vi "一体站流程平行样自动启动.vi"(9 "参数":T1={"是否启用仪器"=FALSE, "CODMn"={"启动测量模式"={"测量模式"=enum."水样测量"}, "确定按钮"=TRUE}, "启动模块"={"氨氮1"=FALSE, "总磷1"=FALSE, " COD1"=FALSE}, "常规启动"=FALSE, "直接启动"=FALSE}) -> ()   [LabVIEW 2016, in "质控单元.lvlib"]
uses:
  PLC/PLC.lvlib
panel:
  out "COD平行样测完标志":bool
  out "氨氮总磷平行样测完标志":bool
  out "枚举 2":enum16{"初始化", "采配水启动", "等待", "配水", "排水", "结束"}(ring)
  out "枚举":enum16{"初始化", "采配水启动", "等待", "配水", "排水", "结束"}(ring)
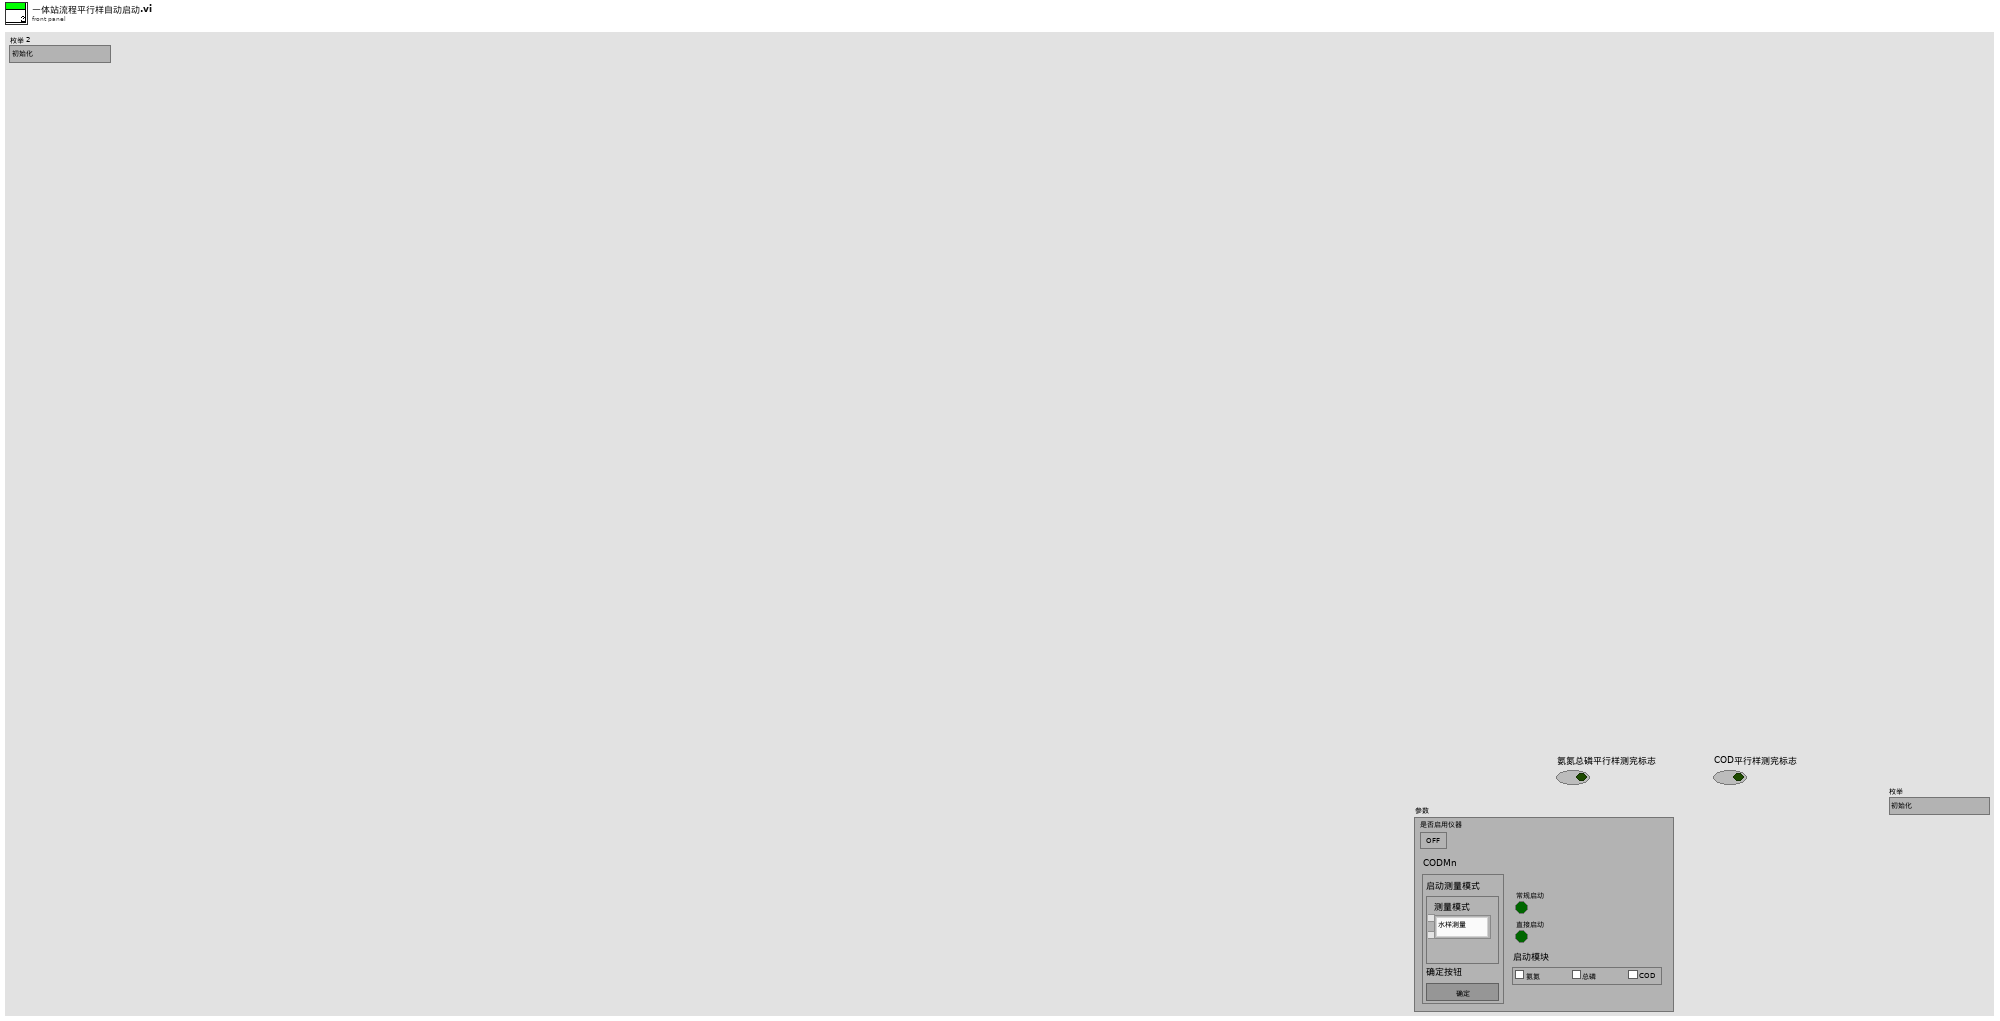
[diagram p1: front panel]
types:
  T1 = cluster{"是否启用仪器":bool, "CODMn":cluster{"启动测量模式":cluster{"测量模式":enum16{"水样测量", "标样核查", "加标回收", "平行样", "校零", "校标"}}, "确定按钮":bool}, "启动模块":cluster{"氨氮1":bool, "总磷1":bool, " COD1":bool}, "常规启动":bool, "直接启动":bool}
  T2 = cluster{"命令":string, cluster{"starting address":u16, "holding register value":u16}}
  T3 = cluster{"R0":i16, "R1":i16, "R2":i16, "R3":i16, "R4":i16, "R5":i16, "R6":i16, "R7":i16, "R8":i16, "R9":i16, "R10":i16, "R11":i16, "R12":i16, "R13":i16, "R14":i16, "R15":i16, "R16":i16, "R17":i16, "R18":i16, "R19":i16, "R20":i16, "R21":i16, "R22":i16, "R23":i16, "R24":i16, "R25":i16, "R26":i16, "R27":i16, "R28":i16, "R29":i16, "R30":i16, "R31":i16, "R32":i16, "R33":i16, "R34":i16}
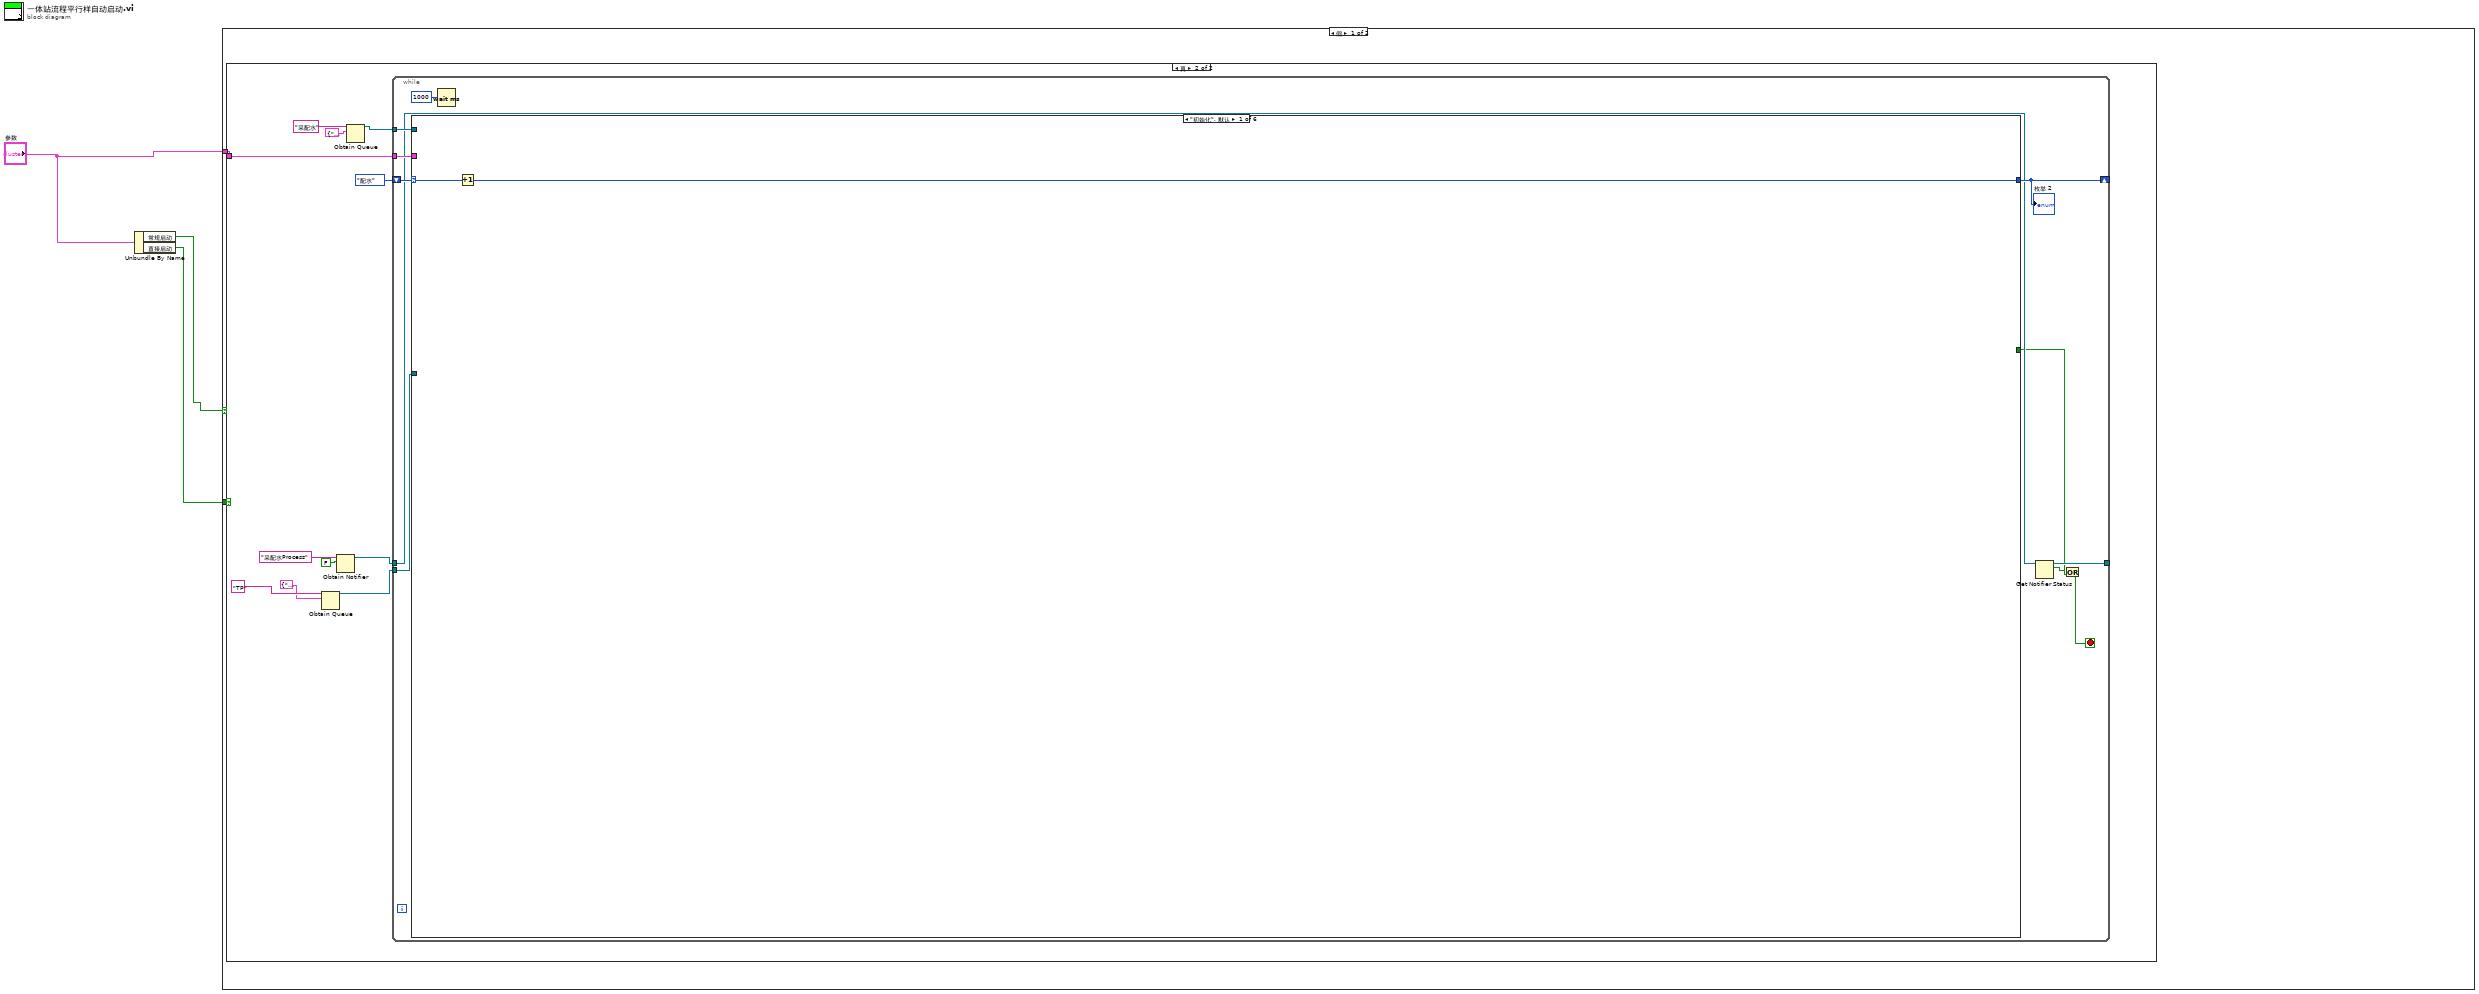
[diagram p0: block diagram]
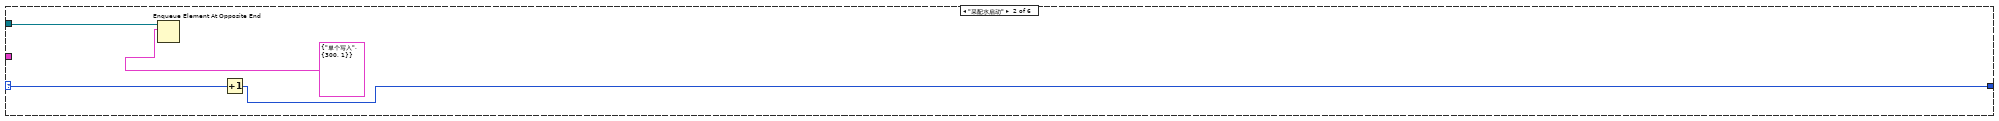
[diagram p3: hidden frame]
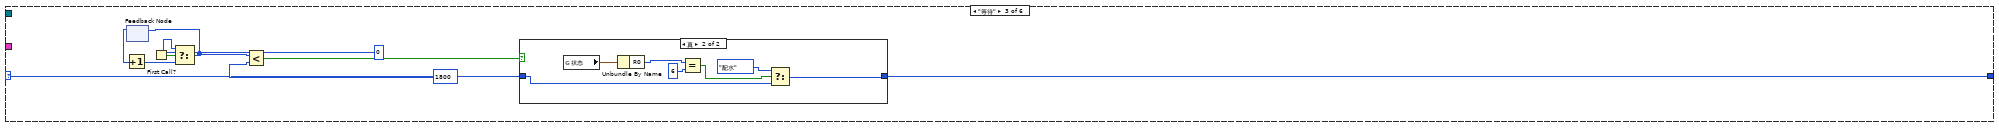
[diagram p4: hidden frame]
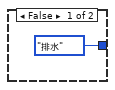
[diagram p5: hidden frame]
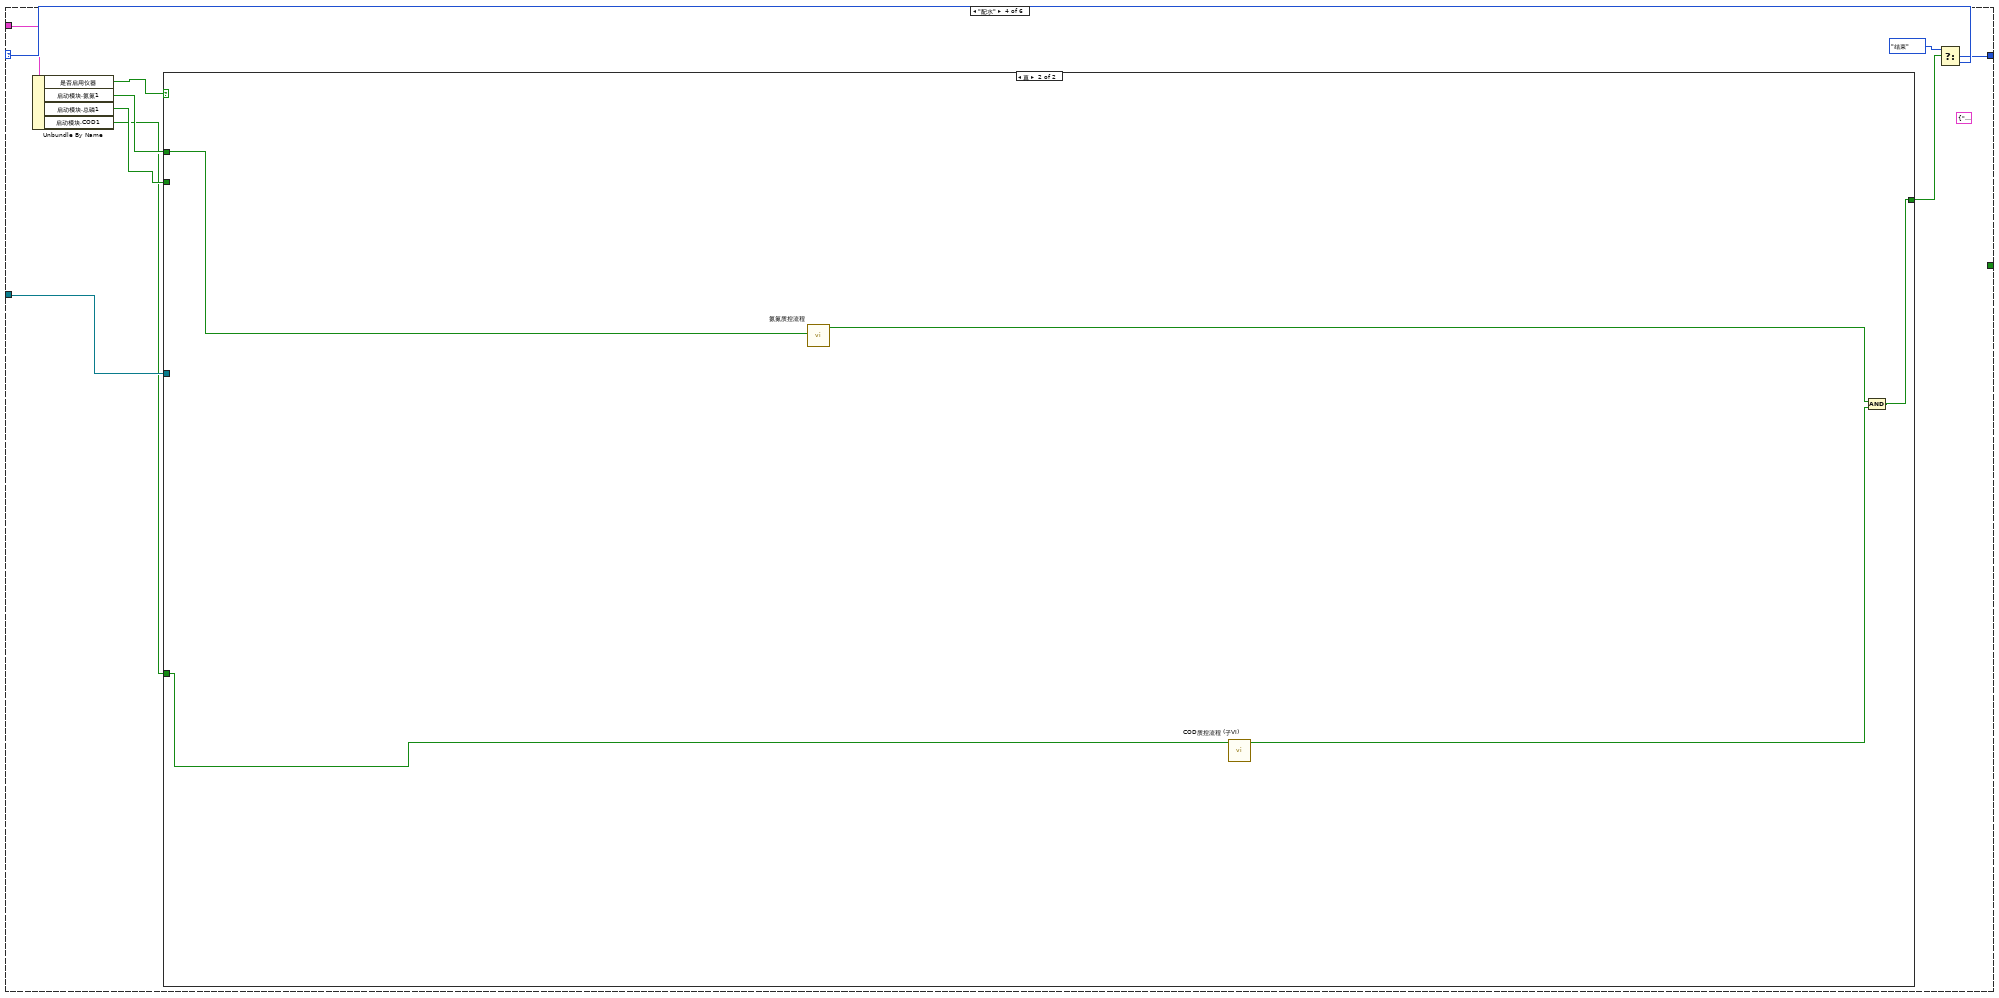
[diagram p6: hidden frame]
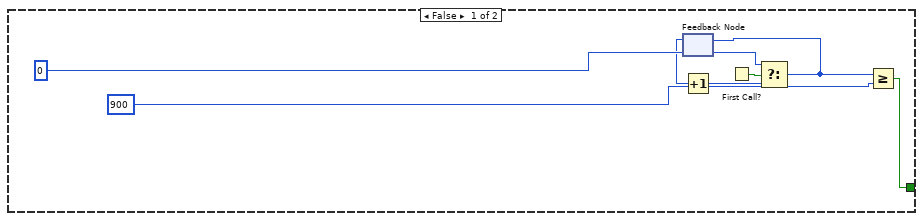
[diagram p7: hidden frame]
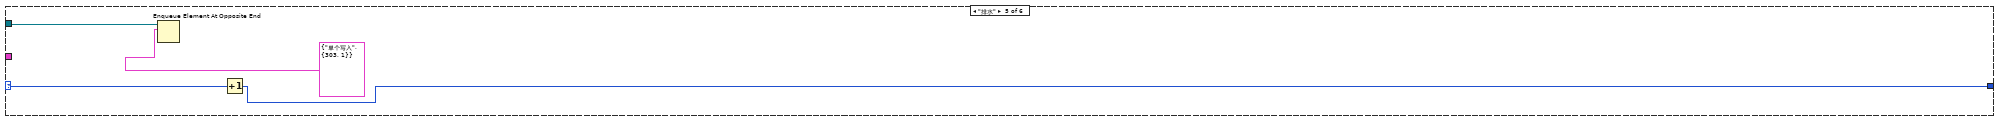
[diagram p8: hidden frame]
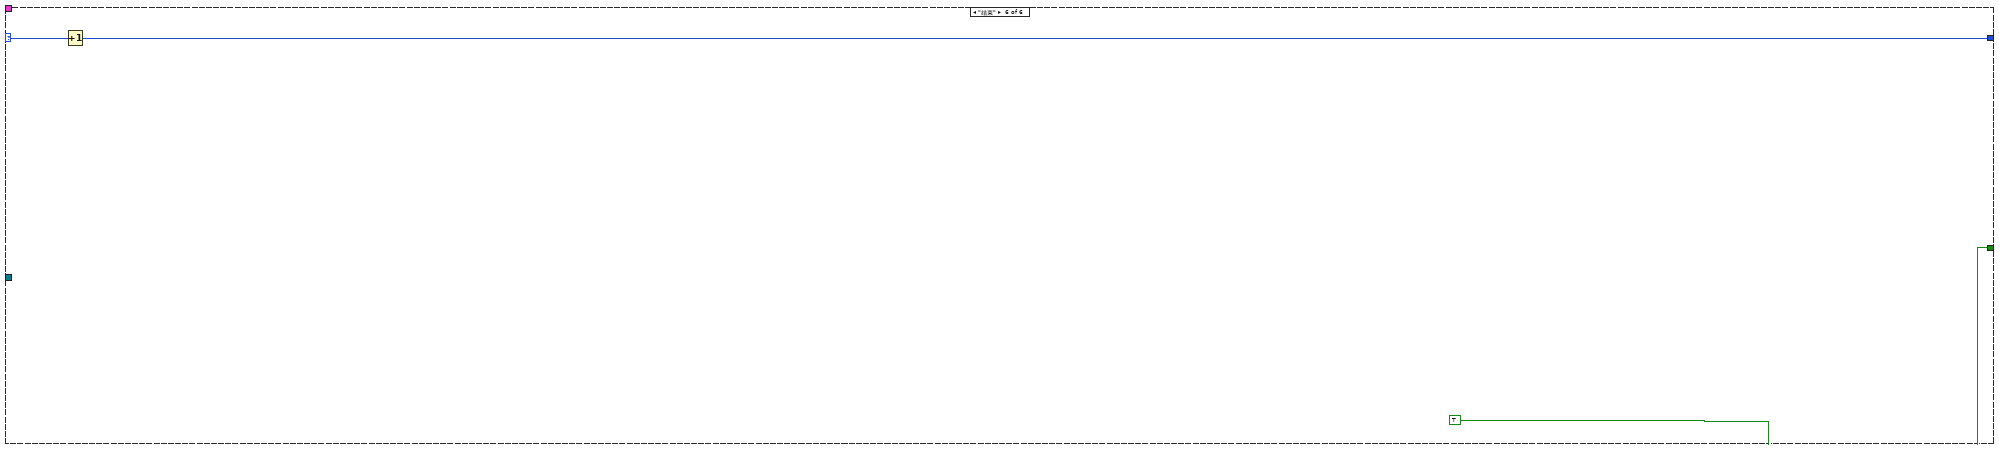
[diagram p9: hidden frame]
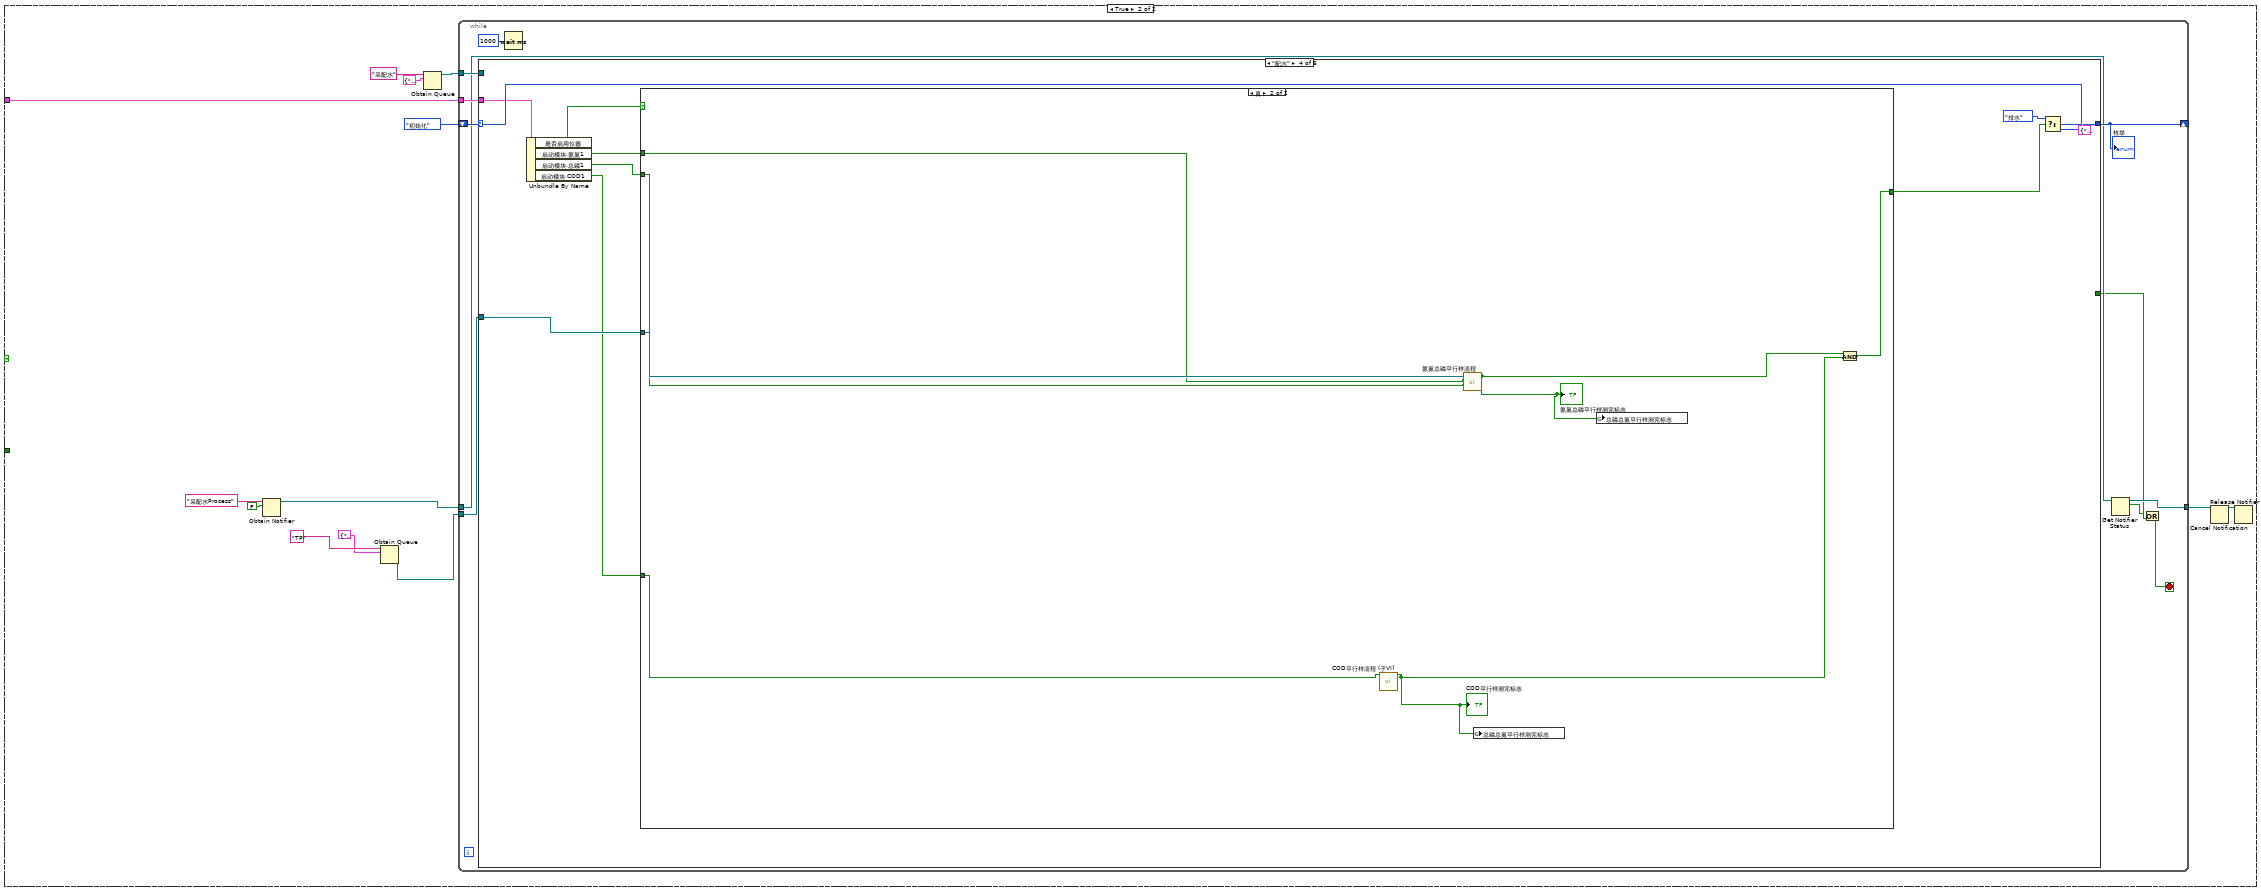
[diagram p10: hidden frame]
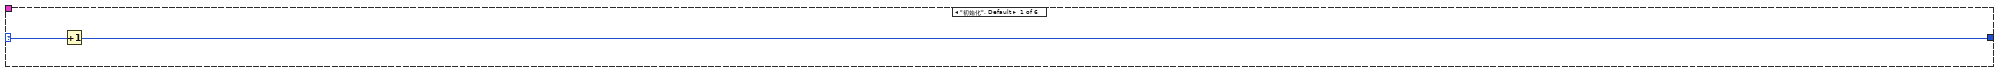
[diagram p11: hidden frame]
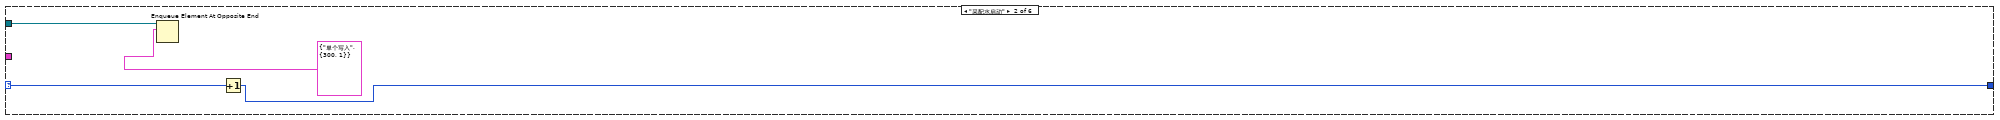
[diagram p12: hidden frame]
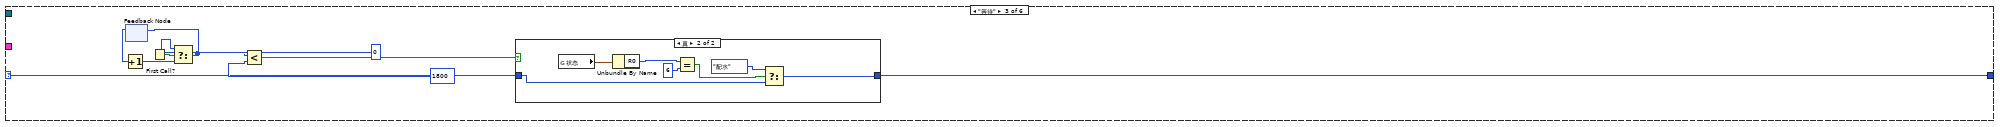
[diagram p13: hidden frame]
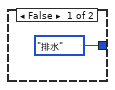
[diagram p14: hidden frame]
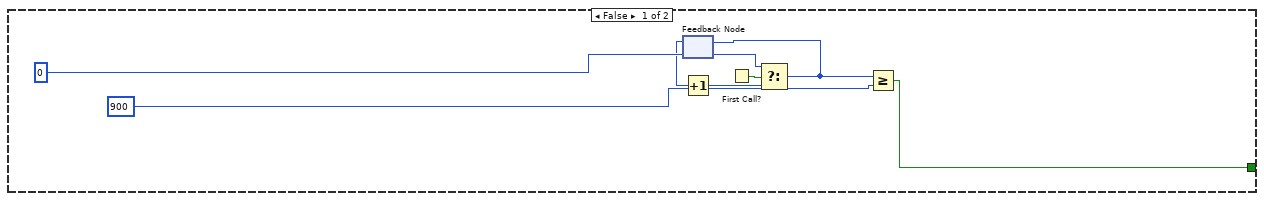
[diagram p15: hidden frame]
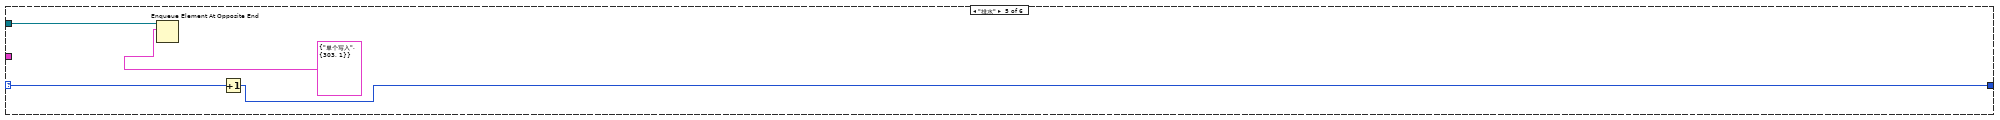
[diagram p16: hidden frame]
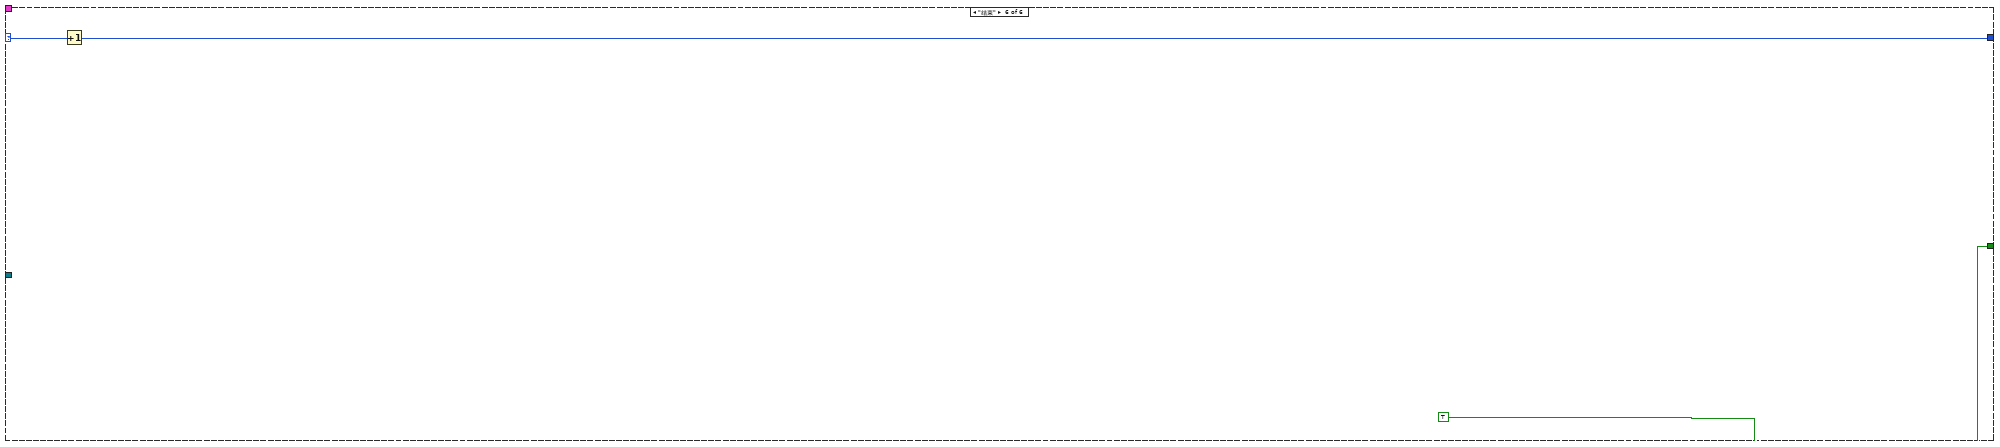
[diagram p17: hidden frame]
diagram:
  n1 = Unbundle By Name("参数") -> ("常规启动"=w2:bool, "直接启动"=w1:bool)
  n2 = case shown="假" w2 {
    tunnel: "参数" -> [w4 w80]
    tunnel: w1 -> [w5 _]
    frame False {
      n3 = case shown="真" w5 {
        tunnel: w4 -> [_ w15]
        frame False {
        }
        frame True {
          n4 = Obtain Queue(name (unnamed)="TP" ("名称（未命名）"), element data type=cluster{"命令":string, "data":variant} {"命令"="", "data"=variant}) -> (queue out=w6:refnum<queue>)  [unwired: 3 in, 2 out]
          n5 = Obtain Notifier(name (unnamed)="采配水Process" ("名称（未命名）"), notification data type=FALSE) -> (notifier out=w9:refnum<notifier>)  [unwired: 2 in, 2 out]
          n6 = Obtain Queue(name (unnamed)="采配水" ("名称（未命名）"), element data type=cluster{"命令":string, "数据":variant} {"命令"="", "数据"=variant}) -> (queue out=w12:refnum<queue>)  [unwired: 3 in, 2 out]
          n7 = while {
            tunnel: w12 -> [w27]
            shift-right: [w25] -> _
            shift-left: enum16{"初始化", "采配水启动", "等待", "配水", "排水", "结束"}."配水" ("枚举") -> [w26]
            tunnel: w6 -> [w23]
            tunnel: w15 -> [w22]
            tunnel: w9 -> [w21]
            tunnel: [w20] -> _
            stop <- w19 stop-if-true
            n8 = case shown="\"初始化\", 默认" w26 {
              selector: w26 -> [w29 w31 w40 w59 w74 w79]
              tunnel: w27 -> [_ w32 _ _ w75 _]
              tunnel: [w28 w30 w39 w58 w73 w78] -> w25
              tunnel: [_ _ _ _ _ TRUE] -> w18
              tunnel: w23 -> [_ _ _ w57 _ _]
              tunnel: w22 -> [_ _ _ w54 _ _]
              frame "初始化", Default {
                n9 = Increment(x=w29) -> (x+1=w28:enum16{"初始化", "采配水启动", "等待", "配水", "排水", "结束"})
              }
              frame "采配水启动" {
                n10 = Enqueue Element At Opposite End(queue=w32, element=T2 {"命令"="单个写入", {"starting address"=300, "holding register value"=1}} ("元素")) -> ()  [unwired: 2 in, 3 out]
                n11 = Increment(x=w31) -> (x+1=w30:enum16{"初始化", "采配水启动", "等待", "配水", "排水", "结束"})
              }
              frame "等待" {
                n12 = feedback #1() -> (w36:i32)  [unwired: 1 in]
                n13 = Increment(x=w36) -> (x+1=w35:i32)
                n14 = First Call?() -> (First Call?: T/F=w37:bool)
                n15 = Select(t=0, s=w37, f=w35) -> (s? t:f=w34:i32)
                n16 = feedback-in #1(w34) -> ()
                n17 = Less?(x=w34, y=1800) -> (x < y?=w41:bool)
                n18 = case shown="真" w41 {
                  tunnel: w40 -> [_ w45]
                  tunnel: [enum16{"初始化", "采配水启动", "等待", "配水", "排水", "结束"}."排水" ("枚举") w44] -> w39
                  frame False {
                  }
                  frame True {
                    n19 = global read "采配水全局变量.vi" "状态"() -> (w50:T3)
                    n20 = Unbundle By Name(w50) -> ("R0"=w49:i16)
                    n21 = Equal?(x=w49, y=i16 6) -> (x = y?=w47:bool)
                    n22 = Select(t=enum16{"初始化", "采配水启动", "等待", "配水", "排水", "结束"}."配水" ("枚举"), s=w47, f=w45) -> (s? t:f=w44:enum16{"初始化", "采配水启动", "等待", "配水", "排水", "结束"})
                  }
                }
              }
              frame "配水" {
                (unwired) cluster{"命令":string, "data":variant} {"命令"="启动", "data"=variant(cluster{"站号":u16, "控制命令输出":u16[]} {"站号"=1, "控制命令输出"=[256, 0]})} ("元素")
                n23 = Unbundle By Name(w54) -> ("是否启用仪器"=w56:bool, "启动模块.氨氮1"=w52:bool, "启动模块.总磷1"=w53:bool, "启动模块.COD1"=w51:bool)
                n24 = case shown="真" w56 {
                  tunnel: w57 -> [_ _]
                  tunnel: [w61 w72] -> w55
                  tunnel: w53 -> [_ _]
                  tunnel: w52 -> [_ w70]
                  tunnel: w51 -> [_ w69]
                  frame False {
                    n25 = feedback #2() -> (w65:i32)  [unwired: 1 in]
                    n26 = Increment(x=w65) -> (x+1=w64:i32)
                    n27 = First Call?() -> (First Call?: T/F=w66:bool)
                    n28 = Select(t=0, s=w66, f=w64) -> (s? t:f=w62:i32)
                    n29 = feedback-in #2(w62) -> ()
                    n30 = Greater Or Equal?(x=w62, y=900) -> (x >= y?=w61:bool)
                  }
                  frame True {
                    n31 = call "氨氮质控流程.vi"("氨氮"=w70) -> ("布尔"=w71:bool)  [unwired: 9 in, 1 out]
                    n32 = call "COD质控流程 (子VI).vi"("COD"=w69) -> ("布尔"=w68:bool)  [unwired: 9 in, 1 out]
                    n33 = And(x=w71, y=w68) -> (x .and. y?=w72:bool)
                  }
                }
                n34 = Select(t=enum16{"初始化", "采配水启动", "等待", "配水", "排水", "结束"}."结束" ("枚举"), s=w55, f=w59) -> (s? t:f=w58:enum16{"初始化", "采配水启动", "等待", "配水", "排水", "结束"})
              }
              frame "排水" {
                n35 = Enqueue Element At Opposite End(queue=w75, element=T2 {"命令"="单个写入", {"starting address"=303, "holding register value"=1}} ("元素")) -> ()  [unwired: 2 in, 3 out]
                n36 = Increment(x=w74) -> (x+1=w73:enum16{"初始化", "采配水启动", "等待", "配水", "排水", "结束"})
              }
              frame "结束" {
                n37 = Increment(x=w79) -> (x+1=w78:enum16{"初始化", "采配水启动", "等待", "配水", "排水", "结束"})
              }
            }
            "枚举 2" <- w25
            n38 = Wait (ms)(milliseconds to wait=u32 1000 ("等待时间（毫秒）")) -> ()  [unwired: 1 out]
            n39 = Get Notifier Status(notifier=w21) -> (notifier out=w20:refnum<notifier>, current notification=w17:bool)  [unwired: 1 in, 3 out]
            n40 = Or(x=w17, y=w18) -> (x .or. y?=w19:bool)
          }
        }
      }
    }
    frame True {
      n41 = Obtain Notifier(name (unnamed)="采配水Process" ("名称（未命名）"), notification data type=FALSE) -> (notifier out=w83:refnum<notifier>)  [unwired: 2 in, 2 out]
      n42 = Obtain Queue(name (unnamed)="TP" ("名称（未命名）"), element data type=cluster{"命令":string, "data":variant} {"命令"="", "data"=variant}) -> (queue out=w86:refnum<queue>)  [unwired: 3 in, 2 out]
      n43 = Obtain Queue(name (unnamed)="采配水" ("名称（未命名）"), element data type=cluster{"命令":string, "数据":variant} {"命令"="", "数据"=variant}) -> (queue out=w90:refnum<queue>)  [unwired: 3 in, 2 out]
      n44 = while {
        tunnel: w90 -> [w103]
        shift-right: [w101] -> _
        shift-left: enum16{"初始化", "采配水启动", "等待", "配水", "排水", "结束"}."初始化" ("枚举") -> [w102]
        tunnel: w86 -> [w99]
        tunnel: w80 -> [w98]
        tunnel: w83 -> [w97]
        tunnel: [w96] -> w82
        stop <- w95 stop-if-true
        n45 = case shown="\"配水\"" w102 {
          selector: w102 -> [w105 w107 w116 w135 w152 w157]
          tunnel: w103 -> [_ w108 _ _ w153 _]
          tunnel: [w104 w106 w115 w134 w151 w156] -> w101
          tunnel: [_ _ _ _ _ TRUE] -> w94
          tunnel: w99 -> [_ _ _ w133 _ _]
          tunnel: w98 -> [_ _ _ w130 _ _]
          frame "初始化", Default {
            n46 = Increment(x=w105) -> (x+1=w104:enum16{"初始化", "采配水启动", "等待", "配水", "排水", "结束"})
          }
          frame "采配水启动" {
            n47 = Enqueue Element At Opposite End(queue=w108, element=T2 {"命令"="单个写入", {"starting address"=300, "holding register value"=1}} ("元素")) -> ()  [unwired: 2 in, 3 out]
            n48 = Increment(x=w107) -> (x+1=w106:enum16{"初始化", "采配水启动", "等待", "配水", "排水", "结束"})
          }
          frame "等待" {
            n49 = feedback #3() -> (w112:i32)  [unwired: 1 in]
            n50 = Increment(x=w112) -> (x+1=w111:i32)
            n51 = First Call?() -> (First Call?: T/F=w113:bool)
            n52 = Select(t=0, s=w113, f=w111) -> (s? t:f=w110:i32)
            n53 = feedback-in #3(w110) -> ()
            n54 = Less?(x=w110, y=1800) -> (x < y?=w117:bool)
            n55 = case shown="真" w117 {
              tunnel: w116 -> [_ w121]
              tunnel: [enum16{"初始化", "采配水启动", "等待", "配水", "排水", "结束"}."排水" ("枚举") w120] -> w115
              frame False {
              }
              frame True {
                n56 = global read "采配水全局变量.vi" "状态"() -> (w126:T3)
                n57 = Unbundle By Name(w126) -> ("R0"=w125:i16)
                n58 = Equal?(x=w125, y=i16 6) -> (x = y?=w123:bool)
                n59 = Select(t=enum16{"初始化", "采配水启动", "等待", "配水", "排水", "结束"}."配水" ("枚举"), s=w123, f=w121) -> (s? t:f=w120:enum16{"初始化", "采配水启动", "等待", "配水", "排水", "结束"})
              }
            }
          }
          frame "配水" {
            (unwired) cluster{"命令":string, "data":variant} {"命令"="启动", "data"=variant(cluster{"站号":u16, "控制命令输出":u16[]} {"站号"=1, "控制命令输出"=[256, 0]})} ("元素")
            n60 = Unbundle By Name(w130) -> ("是否启用仪器"=w132:bool, "启动模块.氨氮1"=w128:bool, "启动模块.总磷1"=w129:bool, "启动模块.COD1"=w127:bool)
            n61 = case shown="真" w132 {
              tunnel: w133 -> [_ w150]
              tunnel: [w137 w147] -> w131
              tunnel: w129 -> [_ w148]
              tunnel: w128 -> [_ w149]
              tunnel: w127 -> [_ w146]
              frame False {
                n62 = feedback #4() -> (w141:i32)  [unwired: 1 in]
                n63 = Increment(x=w141) -> (x+1=w140:i32)
                n64 = First Call?() -> (First Call?: T/F=w142:bool)
                n65 = Select(t=0, s=w142, f=w140) -> (s? t:f=w138:i32)
                n66 = feedback-in #4(w138) -> ()
                n67 = Greater Or Equal?(x=w138, y=900) -> (x >= y?=w137:bool)
              }
              frame True {
                n68 = call "COD平行样流程 (子VI).vi"("COD1"=w146) -> ("布尔"=w144:bool)  [unwired: 10 in]
                "COD平行样测完标志" <- w144
                n69 = call "氨氮总磷平行样流程.vi"("总磷1"=w148, "氨氮1"=w149, "队列输入"=w150) -> ("布尔"=w145:bool)  [unwired: 8 in]
                "氨氮总磷平行样测完标志" <- w145
                n70 = global write "质控测完标志全局 1.vi" "总磷总氮平行样测完标志"(w144) -> ()
                n71 = global write "质控测完标志全局 1.vi" "总磷总氮平行样测完标志"(w145) -> ()
                n72 = And(x=w145, y=w144) -> (x .and. y?=w147:bool)
              }
            }
            n73 = Select(t=enum16{"初始化", "采配水启动", "等待", "配水", "排水", "结束"}."排水" ("枚举"), s=w131, f=w135) -> (s? t:f=w134:enum16{"初始化", "采配水启动", "等待", "配水", "排水", "结束"})
          }
          frame "排水" {
            n74 = Enqueue Element At Opposite End(queue=w153, element=T2 {"命令"="单个写入", {"starting address"=303, "holding register value"=1}} ("元素")) -> ()  [unwired: 2 in, 3 out]
            n75 = Increment(x=w152) -> (x+1=w151:enum16{"初始化", "采配水启动", "等待", "配水", "排水", "结束"})
          }
          frame "结束" {
            n76 = Increment(x=w157) -> (x+1=w156:enum16{"初始化", "采配水启动", "等待", "配水", "排水", "结束"})
          }
        }
        "枚举" <- w101
        n77 = Wait (ms)(milliseconds to wait=u32 1000 ("等待时间（毫秒）")) -> ()  [unwired: 1 out]
        n78 = Get Notifier Status(notifier=w97) -> (notifier out=w96:refnum<notifier>, current notification=w93:bool)  [unwired: 1 in, 3 out]
        n79 = Or(x=w93, y=w94) -> (x .or. y?=w95:bool)
      }
      n80 = Cancel Notification(0:w82) -> (8:w81:refnum<notifier>)  [unwired: 1 in, 2 out]
      n81 = Release Notifier(notifier=w81) -> ()  [unwired: 2 in, 3 out]
    }
  }
